vi "new report subVI.vi"(0 "report in":refnum<class "NI_Word.lvclass">, 1 "window state (normal)":T1(ring)=enum."normal", 5 "display alerts? (F)":bool, 7 "template (empty)":path, 9 "machine name (empty)":string, 11 "error in (no error)":errorcluster) -> (4 "report out":refnum<class "NI_Word.lvclass">, 15 "error out":errorcluster)   [LabVIEW 2015, in "NI_Word.lvclass"]
uses:
  <vilib>/Utility/NIReport.llb/Word/NI_Word.lvclass
  <vilib>/Utility/NIReport.llb/Word/NI_Word.lvclass/NI_Word.ctl
  <vilib>/addons/_office/NI_ReportGenerationToolkit.lvlib
  <vilib>/Utility/NIReport.llb/NI_ReportGenerationCore.lvlib
panel:
  in  "Word._Application":refnum<k7>
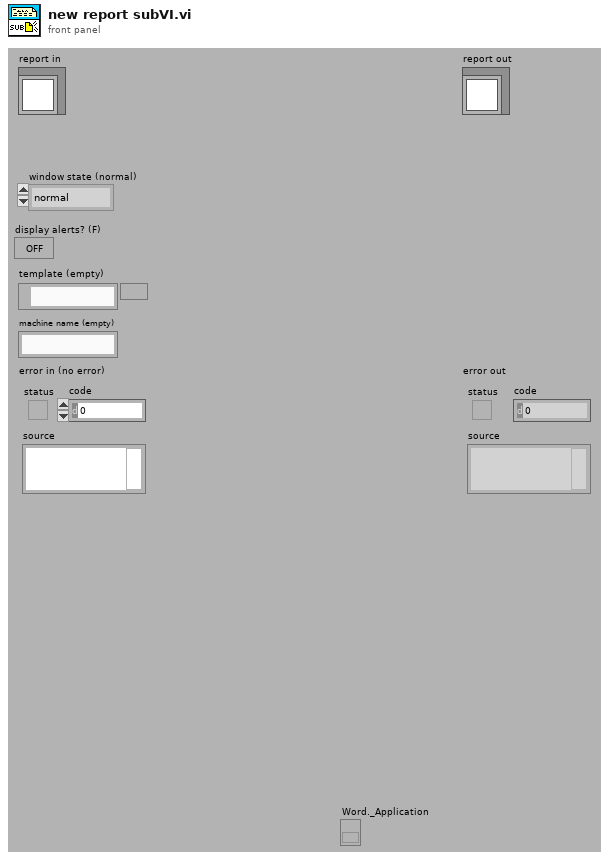
[diagram p1: front panel]
types:
  T1 = enum16{"maximized", "minimized", "normal", "no change"}
  T2 = cluster{"Application":refnum<k7>, "Document":refnum<k7>, "Tables":refnum<k7>, "InlineShapes":refnum<k7>, "Documents":refnum<k7>}
  T3 = typedef "NI_ReportGenerationCore.lvlib/Report Data Members.ctl" = cluster{"font":T4, "from template?":bool}
  T4 = typedef "NI_ReportGenerationCore.lvlib/font.ctl" = cluster{"font name":string, "font size":dbl, "bold":u16, "italic":u16, "underline":u16, "strike through":u16, "font color":u32}
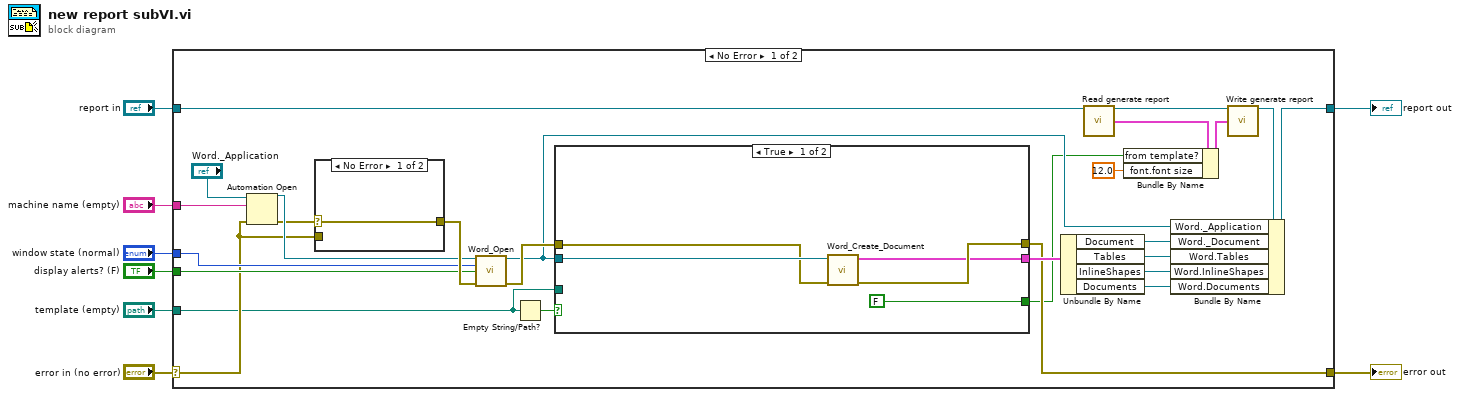
[diagram p0: block diagram]
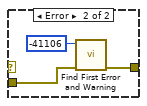
[diagram p2: hidden frame]
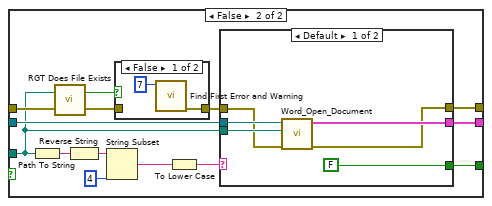
[diagram p3: hidden frame]
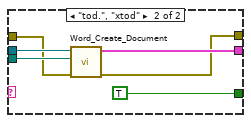
[diagram p5: hidden frame]
diagram:
  n1 = case shown="No Error" "error in (no error)" {
    selector: "error in (no error)" -> [w20 w74]
    tunnel: [w19 w74] -> w7
    tunnel: [w18 w73] -> w5
    tunnel: "report in" -> [w15 w73]
    tunnel: "template (empty)" -> [w17 _]
    tunnel: "machine name (empty)" -> [w23 _]
    tunnel: "display alerts? (F)" -> [w22 _]
    tunnel: "window state (normal)" -> [w21 _]
    frame No Error {
      n2 = Automation Open(machine name=w23, error in (no error)=w20, Automation Refnum="Word._Application") -> (Automation Refnum=w31:refnum<k7>, error out=w30:errorcluster)  [unwired: 1 out]
      n3 = case shown="No Error" w30 {
        selector: w30 -> [w35 _]
        tunnel: [w35 w37] -> w34
        tunnel: w20 -> [_ w36]
        frame No Error {
        }
        frame Error {
          n4 = call <vilib>:"Find First Error and Warning.vi"("error in (no error)"=w36, "error code"=-41106) -> ("error out"=w37:errorcluster)  [unwired: 5 out]
        }
      }
      n5 = call <vilib>:"Word_Open.vi"("word application in"=w31, "window state"=w21, "display alerts?"=w22, "Error in"=w34) -> ("word application out"=w32:refnum<k7>, "Error out"=w33:errorcluster)  [unwired: 10 out]
      n6 = Empty String/Path?(string/path=w17) -> (empty?=w16:bool)
      n7 = case shown="True" w16 {
        tunnel: [w39 w57] -> w24
        tunnel: w32 -> [w42 w52]
        tunnel: w33 -> [w41 w51]
        tunnel: [w40 w56] -> w19
        tunnel: w17 -> [_ w50]
        tunnel: [FALSE w46] -> w10
        frame True {
          n8 = call <vilib>:"Word_Create_Document.vi"("error in"=w41, "word application"=w42) -> ("error out"=w40:errorcluster, "references"=w39:T2)  [unwired: 1 in, 3 out]
        }
        frame False {
          n9 = Path To String(path=w50) -> (string=w55:string)
          n10 = call <vilib>:"RGT Does File Exists.vi"("error in (no error)"=w51, "path"=w50) -> ("error out"=w49:errorcluster, "file exists?"=w47:bool)
          n11 = Reverse String(1:w55) -> (0:w54:string)
          n12 = String Subset(string=w54, length (rest)=4 ("length (rest)")) -> (substring=w45:string)  [unwired: 1 out]
          n13 = case shown="False" w47 {
            tunnel: w49 -> [_ w60]
            tunnel: [w58 w60] -> w48
            frame False {
              n14 = call <vilib>:"Find First Error and Warning.vi"("error code"=7) -> ("error out"=w58:errorcluster)  [unwired: 1 in, 5 out]
            }
            frame True {
            }
          }
          n15 = To Lower Case(string=w45) -> (all lower case string=w44:string)
          n16 = case shown="Default" w44 {
            tunnel: [w63 w69] -> w57
            tunnel: w52 -> [w65 w71]
            tunnel: w48 -> [w61 w67]
            tunnel: [w62 w68] -> w56
            tunnel: w50 -> [w64 w70]
            tunnel: [FALSE TRUE] -> w46
            frame Default {
              n17 = call <vilib>:"Word_Open_Document.vi"("error in"=w61, "document path"=w64, "word application"=w65) -> ("error out"=w62:errorcluster, "references"=w63:T2)  [unwired: 3 out]
            }
            frame "tod.", "xtod" {
              n18 = call <vilib>:"Word_Create_Document.vi"("error in"=w67, "Template Path"=w70, "word application"=w71) -> ("error out"=w68:errorcluster, "references"=w69:T2)  [unwired: 3 out]
            }
          }
        }
      }
      n19 = Unbundle By Name(w24) -> ("Document"=w25:refnum<k7>, "Tables"=w26:refnum<k7>, "InlineShapes"=w27:refnum<k7>, "Documents"=w28:refnum<k7>)
      n20 = call-dynamic "Read generate report.vi"("report in"=w15) -> ("report out"=w14:refnum<class "NI_Word.lvclass">, "generate report"=w12:T3)  [unwired: 12 in, 1 out]
      n21 = Bundle By Name(cluster=w12, "from template?"=w10, "font.font size"=12.0) -> (w11:T3)
      n22 = call-dynamic "Write generate report.vi"("report in"=w14, "generate report"=w11) -> ("report out"=w13:refnum<class "NI_Word.lvclass">)  [unwired: 12 in, 1 out]
      n23 = Bundle By Name(cluster=w13, "Word._Application"=w32, "Word._Document"=w25, "Word.Tables"=w26, "Word.InlineShapes"=w27, "Word.Documents"=w28) -> (w18:refnum<class "NI_Word.lvclass">)
    }
    frame Error {
    }
  }
  "error out" <- w7
  "report out" <- w5
